vi "GetDiodeCurrent.vi"(8 "error in (no error)":errorcluster, 11 "Laser Diode Controller in":refnum<class "KLD101.lvclass">) -> (0 "error out":errorcluster, 2 "diodeCurrent":dbl, 3 "Laser Diode Controller out":refnum<class "KLD101.lvclass">)   [LabVIEW 2016, in "Laser Diode Controller.lvlib" / "KLD101.lvclass"]
uses:
  KLD101.lvclass
  KLD101.lvclass/KLD101.ctl
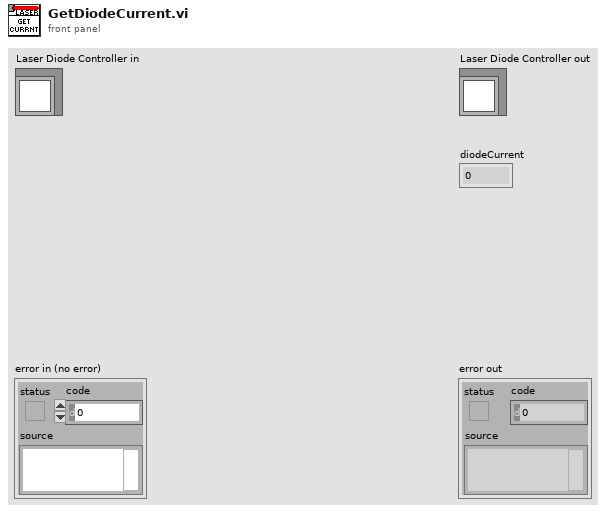
[diagram p1: front panel]
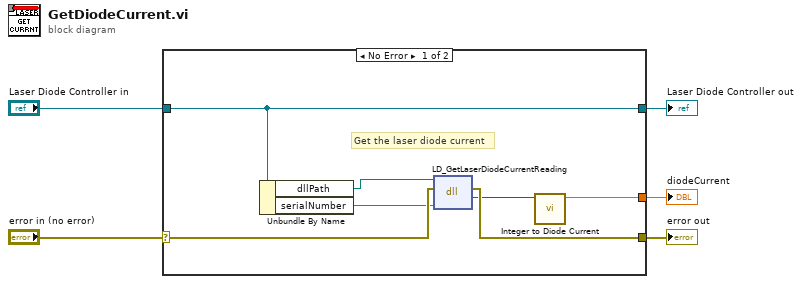
[diagram p0: block diagram]
diagram:
  n1 = case shown="No Error" "error in (no error)" {
    selector: "error in (no error)" -> [w12 w14]
    tunnel: [w11 w14] -> w4
    tunnel: [w9 w13] -> w2
    tunnel: "Laser Diode Controller in" -> [w9 w13]
    tunnel: [w10 _] -> w1
    frame No Error {
      # "Get the laser diode current"
      n2 = Unbundle By Name(w9) -> ("dllPath"=w6:path, "serialNumber"=w8:string)
      n3 = dll-call lib="C:/IDEXX Software/Collimation/data/Thorlabs.MotionControl.KCube.LaserDiode.dll" fn="LD_GetLaserDiodeCurrentReading"(path in=w6, error in=w12, "serialNumber"=w8) -> (error out=w11:errorcluster, "current"=w7:i16)  [unwired: 2 in, 1 out]
      n4 = call "Integer to Diode Current.vi"("Current Int"=w7) -> ("Current (mA)"=w10:dbl)  [unwired: 10 in]
    }
    frame Error {
    }
  }
  "error out" <- w4
  "Laser Diode Controller out" <- w2
  "diodeCurrent" <- w1
